vi "read mouse.vi"(0 "Display State In":T1={"keyboard ref"=refnum, "mouse ref"=refnum, "control refs"={"check mouse"=refnum}, "settings"={"key"=enum."RIGHT", "increment"=0.0}}, 9 "Container State":T4, 11 "error in (no error)":errorcluster) -> (4 "Display State Out":T1={"keyboard ref"=refnum, "mouse ref"=refnum, "control refs"={"check mouse"=refnum}, "settings"={"key"=enum."RIGHT", "increment"=0.0}}, 15 "error out":errorcluster)   [LabVIEW 2010, in "XMouseSlider.xctl"]
uses:
  XMouseSlider.xctl
  <vilib>/_xctls/Container State.ctl
  state.ctl
  control_refs_cluster.ctl
  settings_cluster.ctl
  <vilib>/_xctls/XControlSupport.lvlib
panel:
  # "Add Controls & Indicators that form the parameters of the method here. Hook them to the connector pane. Do not delete the controls & indicators that are already hooked to the connector pane.\n \nTo setup the parameters  for this method, right click on this item in the Project Tree & select \"Configure Method...\"."
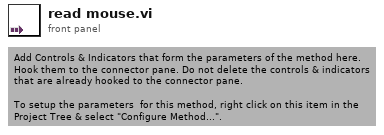
[diagram p1: front panel]
types:
  T1 = typedef "XMouseSlider.xctl/state.ctl" = cluster{"keyboard ref":refnum<k1>, "mouse ref":refnum<k1>, "control refs":T2, "settings":T3}
  T2 = typedef "XMouseSlider.xctl/control_refs_cluster.ctl" = cluster{"check mouse":refnum<vi>}
  T3 = typedef "XMouseSlider.xctl/settings_cluster.ctl" = cluster{"key":enum16{"0", "1", "2", "3", "4", "5", "6", "7", "8", "9", "A", "B", "C", "D", "E", "F", "G", "H", "I", "J", "K", "L", "M", "N", "O", "P", "Q", "R", "S", "T", "U", "V", "W", "X", "Y", "Z", "F1", "F2", "F3", "F4", "F5", "F6", "F7", "F8", "F9", "F10", "F11", "F12", "F13", "F14", "F15", "ADD", "BACK", "BACKSLASH", "CAPITAL", "COMMA", "DECIMAL", "DELETE", "DIVIDE", "DOWN", "END", "EQUALS", "ESCAPE", "GRAVE (`)", "HOME", "INSERT", "LBRACKET", "LCONTROL", "LEFT", "L ALT", "LSHIFT", "LWIN", "MINUS", "MULTIPLY", "NEXT", "NUMLOCK", "NUMPAD_0", "NUMPAD_1", "NUMPAD_2", "NUMPAD_3", "NUMPAD_4", "NUMPAD_5", "NUMPAD_6", "NUMPAD_7", "NUMPAD_8", "NUMPAD_9", "PAUSE", "PERIOD", "PRIOR (PG UP)", "RBRACKET", "RCONTROL", "RETURN", "RIGHT", "R ALT", "RSHIFT", "RWIN", "SCROLL", "SEMICOLON", "SLASH", "SPACE", "SUBTRACT", "TAB", "UP", "ENTER (num pad)", "' (quote)"}, "increment":dbl}
  T4 = typedef "XControlSupport.lvlib/Container State.ctl" = cluster{"Indicator?":bool, "Run Mode?":bool, " Refnum":refnum<vi>}
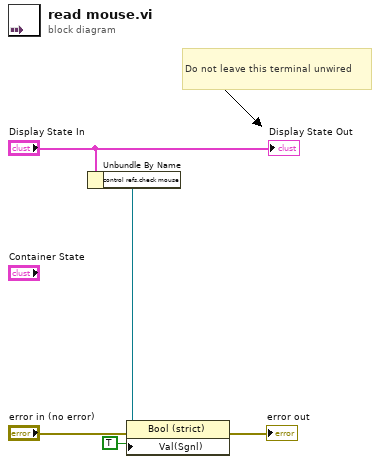
[diagram p0: block diagram]
diagram:
  # "Do not leave this terminal unwired"
  n1 = Unbundle By Name("Display State In") -> ("control refs.check mouse"=w4:refnum<vi>)
  n2 = property class="Bool (strict)"(reference=w4, error in="error in (no error)", "Val(Sgnl)"=TRUE ("Value (Signaling)")) -> (error out=→"error out":errorcluster)  [unwired: 1 out]
  "Display State Out" <- "Display State In"
